vi "PFI-28000-Channel_Get Channel Number.vi"(8 "error in (no error)":errorcluster, 11 "PFI-28000-Channel in":refnum<class "PFI-28000-Channel.lvclass">) -> (0 "error out":errorcluster, 2 "Channel Number":i32, 3 "PFI-28000-Channel out":refnum<class "PFI-28000-Channel.lvclass">)   [LabVIEW 2017, in "PFI-28000-Channel.lvclass"]
uses:
  PFI-28000-Channel.lvclass
  PFI-28000-Channel.lvclass/PFI-28000-Channel.ctl
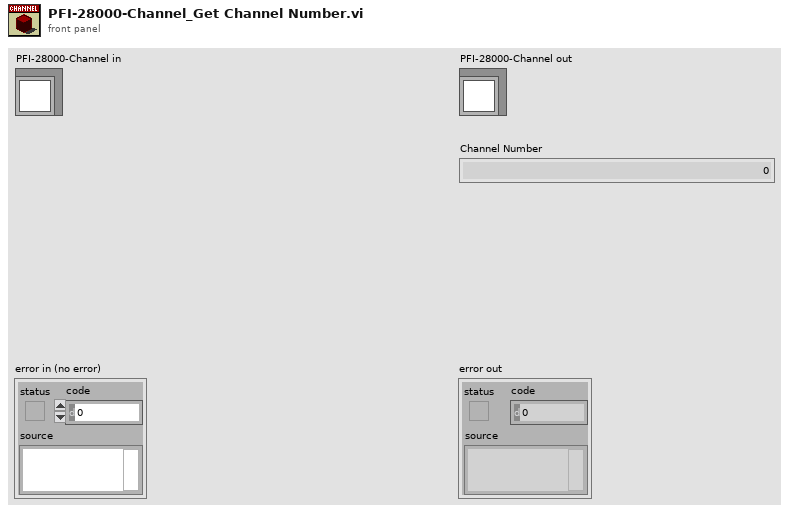
[diagram p1: front panel]
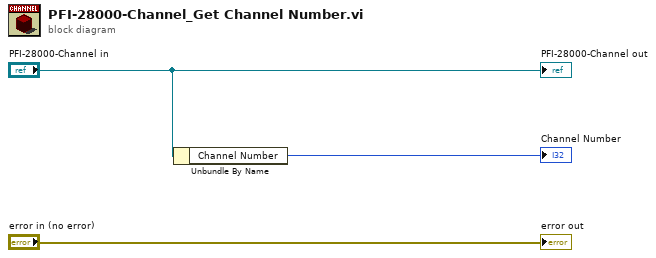
[diagram p0: block diagram]
diagram:
  n1 = Unbundle By Name("PFI-28000-Channel in") -> ("Channel Number"=→"Channel Number":i32)
  "error out" <- "error in (no error)"
  "PFI-28000-Channel out" <- "PFI-28000-Channel in"
